vi "__Test_U8ArrayToData.vi"() -> ()   [LabVIEW 2019, in "Memory Data Access.lvlib"]
uses:
  Memory Data Access.lvlib
panel:
  out "data_Cluster":T1
  out "data_Path":path
  out "data_Str":string
  out "data_DBL":dbl
  out "data_U32":u32
  out "data_I32":i32
  out "data_Waveform":waveform(dbl)
  out "data TimeStamp":timestamp
  out "data_Bool":bool
  out "data_ArrayWav":waveform(dbl)[](array[waveform])
  out "data_ArrayDBL":dbl[](array[numeric])
  out "data_ArrayStr":string[](array[string])
  in  "Enum":T2(ring)
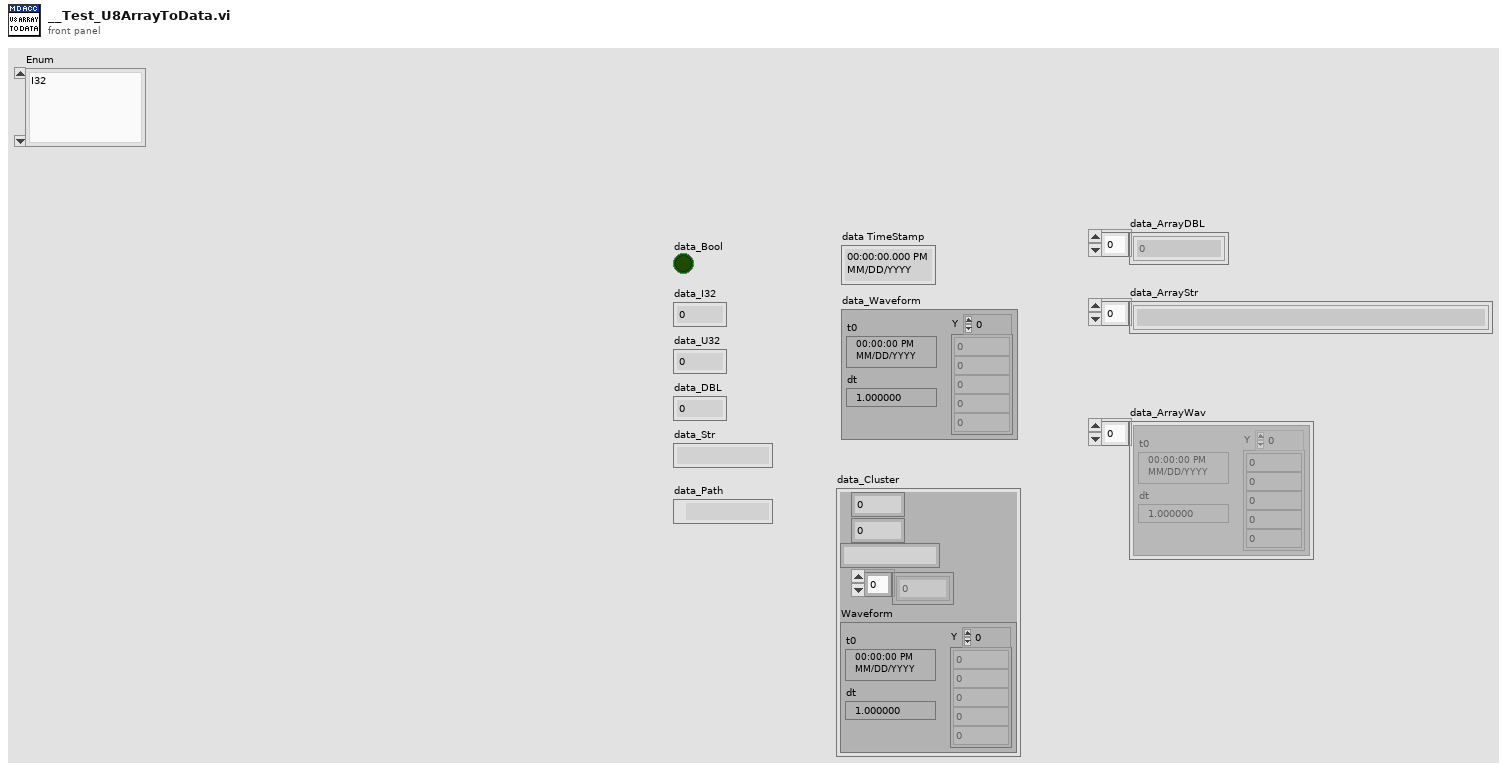
[diagram p1: front panel]
types:
  T1 = cluster{i32, dbl, string, dbl[], "Waveform":waveform(dbl)}
  T2 = enum16{"I32", "U32", "DBL", "String", "Cluster", "Array_Str", "Array_DBL", "Array_Waveform", "Bool", "TimeStamp", "Waveform", "Path"}
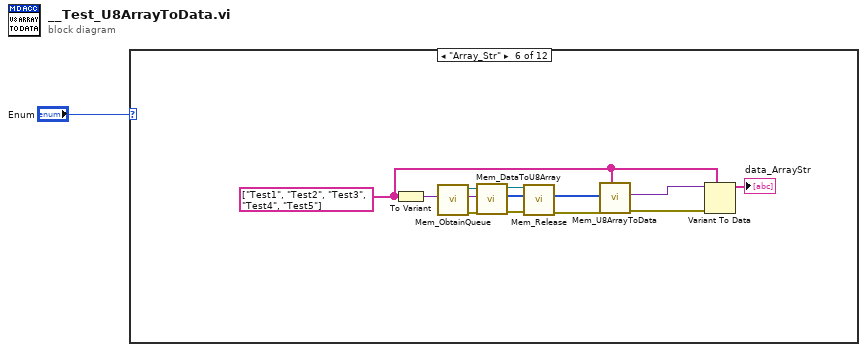
[diagram p0: block diagram]
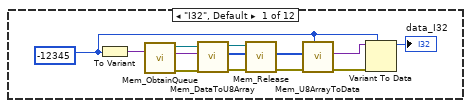
[diagram p2: hidden frame]
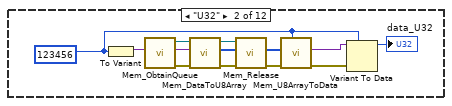
[diagram p3: hidden frame]
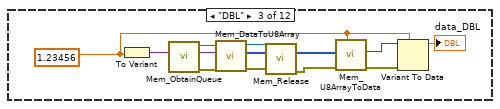
[diagram p4: hidden frame]
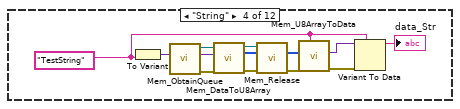
[diagram p5: hidden frame]
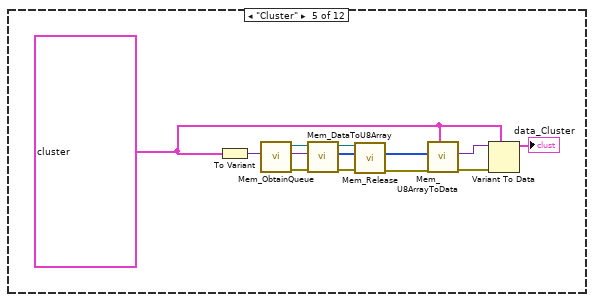
[diagram p6: hidden frame]
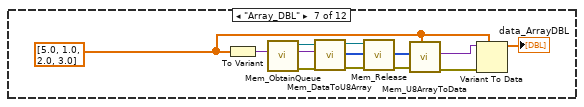
[diagram p7: hidden frame]
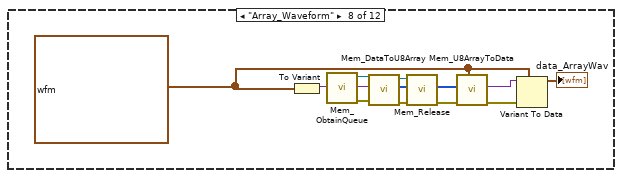
[diagram p8: hidden frame]
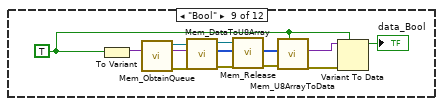
[diagram p9: hidden frame]
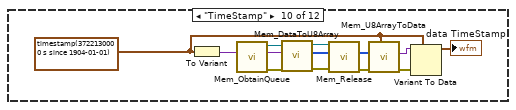
[diagram p10: hidden frame]
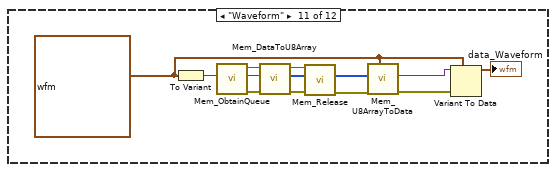
[diagram p11: hidden frame]
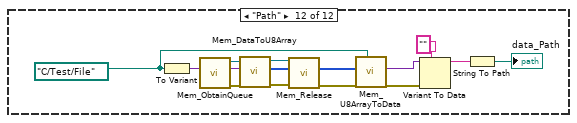
[diagram p12: hidden frame]
diagram:
  n1 = case shown="\"Array_Str\"" "Enum" {
    frame "I32", Default {
      w8 = -12345
      n2 = To Variant(anything=w8) -> (Variant=w12:variant)
      n3 = call "Mem_ObtainQueue.vi"() -> ("error out"=w6:errorcluster, "queue out"=w3:refnum<queue>)  [unwired: 10 in]
      n4 = call "Mem_DataToU8Array.vi"("error in (no error)"=w6, "Payload"=w12, "AddrQueueIn"=w3) -> ("error out"=w5:errorcluster, "ByteArray"=w11:u8[], "AddrQueueOut"=w4:refnum<queue>)  [unwired: 5 in, 1 out]
      n5 = call "Mem_Release.vi"("error in (no error)"=w5, "AddrQueueIn"=w4) -> ("error out"=w2:errorcluster)  [unwired: 9 in]
      n6 = call "Mem_U8ArrayToData.vi"("Type"=w8, "error in (no error)"=w2, "ByteArray"=w11) -> ("error out"=w10:errorcluster, "data"=w9:variant)  [unwired: 5 in, 2 out]
      n7 = Variant To Data(error in=w10, type=w8, Variant=w9) -> (data=→"data_I32":i32)  [unwired: 1 out]
    }
    frame "U32" {
      w19 = u32 123456
      n8 = To Variant(anything=w19) -> (Variant=w23:variant)
      n9 = call "Mem_ObtainQueue.vi"() -> ("error out"=w17:errorcluster, "queue out"=w16:refnum<queue>)  [unwired: 10 in]
      n10 = call "Mem_DataToU8Array.vi"("error in (no error)"=w17, "Payload"=w23, "AddrQueueIn"=w16) -> ("error out"=w15:errorcluster, "ByteArray"=w22:u8[], "AddrQueueOut"=w14:refnum<queue>)  [unwired: 5 in, 1 out]
      n11 = call "Mem_Release.vi"("error in (no error)"=w15, "AddrQueueIn"=w14) -> ("error out"=w13:errorcluster)  [unwired: 9 in]
      n12 = call "Mem_U8ArrayToData.vi"("Type"=w19, "error in (no error)"=w13, "ByteArray"=w22) -> ("error out"=w20:errorcluster, "data"=w21:variant)  [unwired: 5 in, 2 out]
      n13 = Variant To Data(error in=w20, type=w19, Variant=w21) -> (data=→"data_U32":u32)  [unwired: 1 out]
    }
    frame "DBL" {
      w30 = 1.23456
      n14 = To Variant(anything=w30) -> (Variant=w34:variant)
      n15 = call "Mem_ObtainQueue.vi"() -> ("error out"=w28:errorcluster, "queue out"=w27:refnum<queue>)  [unwired: 10 in]
      n16 = call "Mem_DataToU8Array.vi"("error in (no error)"=w28, "Payload"=w34, "AddrQueueIn"=w27) -> ("error out"=w26:errorcluster, "ByteArray"=w33:u8[], "AddrQueueOut"=w25:refnum<queue>)  [unwired: 5 in, 1 out]
      n17 = call "Mem_Release.vi"("error in (no error)"=w26, "AddrQueueIn"=w25) -> ("error out"=w24:errorcluster)  [unwired: 9 in]
      n18 = call "Mem_U8ArrayToData.vi"("Type"=w30, "error in (no error)"=w24, "ByteArray"=w33) -> ("error out"=w32:errorcluster, "data"=w31:variant)  [unwired: 5 in, 2 out]
      n19 = Variant To Data(error in=w32, type=w30, Variant=w31) -> (data=→"data_DBL":dbl)  [unwired: 1 out]
    }
    frame "String" {
      w41 = "TestString"
      n20 = To Variant(anything=w41) -> (Variant=w45:variant)
      n21 = call "Mem_ObtainQueue.vi"() -> ("error out"=w39:errorcluster, "queue out"=w38:refnum<queue>)  [unwired: 10 in]
      n22 = call "Mem_DataToU8Array.vi"("error in (no error)"=w39, "Payload"=w45, "AddrQueueIn"=w38) -> ("error out"=w37:errorcluster, "ByteArray"=w44:u8[], "AddrQueueOut"=w36:refnum<queue>)  [unwired: 5 in, 1 out]
      n23 = call "Mem_Release.vi"("error in (no error)"=w37, "AddrQueueIn"=w36) -> ("error out"=w35:errorcluster)  [unwired: 9 in]
      n24 = call "Mem_U8ArrayToData.vi"("Type"=w41, "error in (no error)"=w35, "ByteArray"=w44) -> ("error out"=w43:errorcluster, "data"=w42:variant)  [unwired: 5 in, 2 out]
      n25 = Variant To Data(error in=w43, type=w41, Variant=w42) -> (data=→"data_Str":string)  [unwired: 1 out]
    }
    frame "Cluster" {
      w52 = T1 {1245, 1.2345, "TestString", [0.0, 1.0, 2.0, 3.0], "Waveform"={"t0"=timestamp(3722126400 s since 1904-01-01), "dt"=1.0, "Y"=[1.0, 2.0, 3.0, 4.0]}}
      n26 = To Variant(anything=w52) -> (Variant=w56:variant)
      n27 = call "Mem_ObtainQueue.vi"() -> ("error out"=w50:errorcluster, "queue out"=w49:refnum<queue>)  [unwired: 10 in]
      n28 = call "Mem_DataToU8Array.vi"("error in (no error)"=w50, "Payload"=w56, "AddrQueueIn"=w49) -> ("error out"=w47:errorcluster, "ByteArray"=w55:u8[], "AddrQueueOut"=w48:refnum<queue>)  [unwired: 5 in, 1 out]
      n29 = call "Mem_Release.vi"("error in (no error)"=w47, "AddrQueueIn"=w48) -> ("error out"=w46:errorcluster)  [unwired: 9 in]
      n30 = call "Mem_U8ArrayToData.vi"("Type"=w52, "error in (no error)"=w46, "ByteArray"=w55) -> ("error out"=w53:errorcluster, "data"=w54:variant)  [unwired: 5 in, 2 out]
      n31 = Variant To Data(error in=w53, type=w52, Variant=w54) -> (data=→"data_Cluster":T1)  [unwired: 1 out]
    }
    frame "Array_Str" {
      w64 = string[] ["Test1", "Test2", "Test3", "Test4", "Test5"]
      n32 = To Variant(anything=w64) -> (Variant=w67:variant)
      n33 = call "Mem_ObtainQueue.vi"() -> ("error out"=w61:errorcluster, "queue out"=w60:refnum<queue>)  [unwired: 10 in]
      n34 = call "Mem_DataToU8Array.vi"("error in (no error)"=w61, "Payload"=w67, "AddrQueueIn"=w60) -> ("error out"=w59:errorcluster, "ByteArray"=w66:u8[], "AddrQueueOut"=w57:refnum<queue>)  [unwired: 5 in, 1 out]
      n35 = call "Mem_Release.vi"("error in (no error)"=w59, "AddrQueueIn"=w57) -> ("error out"=w58:errorcluster)  [unwired: 9 in]
      n36 = call "Mem_U8ArrayToData.vi"("Type"=w64, "error in (no error)"=w58, "ByteArray"=w66) -> ("error out"=w62:errorcluster, "data"=w65:variant)  [unwired: 5 in, 2 out]
      n37 = Variant To Data(error in=w62, type=w64, Variant=w65) -> (data=→"data_ArrayStr":string[])  [unwired: 1 out]
    }
    frame "Array_DBL" {
      w74 = dbl[] [5.0, 1.0, 2.0, 3.0]
      n38 = To Variant(anything=w74) -> (Variant=w78:variant)
      n39 = call "Mem_ObtainQueue.vi"() -> ("error out"=w72:errorcluster, "queue out"=w70:refnum<queue>)  [unwired: 10 in]
      n40 = call "Mem_DataToU8Array.vi"("error in (no error)"=w72, "Payload"=w78, "AddrQueueIn"=w70) -> ("error out"=w71:errorcluster, "ByteArray"=w77:u8[], "AddrQueueOut"=w69:refnum<queue>)  [unwired: 5 in, 1 out]
      n41 = call "Mem_Release.vi"("error in (no error)"=w71, "AddrQueueIn"=w69) -> ("error out"=w68:errorcluster)  [unwired: 9 in]
      n42 = call "Mem_U8ArrayToData.vi"("Type"=w74, "error in (no error)"=w68, "ByteArray"=w77) -> ("error out"=w75:errorcluster, "data"=w76:variant)  [unwired: 5 in, 2 out]
      n43 = Variant To Data(error in=w75, type=w74, Variant=w76) -> (data=→"data_ArrayDBL":dbl[])  [unwired: 1 out]
    }
    frame "Array_Waveform" {
      w85 = waveform(dbl)[] [{"t0"=timestamp(3705278400 s since 1904-01-01), "dt"=1.0, "Y"=[1.0, 2.0, 3.0]}, {"t0"=timestamp(3705278400 s since 1904-01-01), "dt"=1.0, "Y"=[4.0, 5.0, 6.0]}]
      n44 = To Variant(anything=w85) -> (Variant=w89:variant)
      n45 = call "Mem_ObtainQueue.vi"() -> ("error out"=w83:errorcluster, "queue out"=w81:refnum<queue>)  [unwired: 10 in]
      n46 = call "Mem_DataToU8Array.vi"("error in (no error)"=w83, "Payload"=w89, "AddrQueueIn"=w81) -> ("error out"=w82:errorcluster, "ByteArray"=w88:u8[], "AddrQueueOut"=w80:refnum<queue>)  [unwired: 5 in, 1 out]
      n47 = call "Mem_Release.vi"("error in (no error)"=w82, "AddrQueueIn"=w80) -> ("error out"=w79:errorcluster)  [unwired: 9 in]
      n48 = call "Mem_U8ArrayToData.vi"("Type"=w85, "error in (no error)"=w79, "ByteArray"=w88) -> ("error out"=w87:errorcluster, "data"=w86:variant)  [unwired: 5 in, 2 out]
      n49 = Variant To Data(error in=w87, type=w85, Variant=w86) -> (data=→"data_ArrayWav":waveform(dbl)[])  [unwired: 1 out]
    }
    frame "Bool" {
      w96 = TRUE
      n50 = To Variant(anything=w96) -> (Variant=w100:variant)
      n51 = call "Mem_ObtainQueue.vi"() -> ("error out"=w94:errorcluster, "queue out"=w93:refnum<queue>)  [unwired: 10 in]
      n52 = call "Mem_DataToU8Array.vi"("error in (no error)"=w94, "Payload"=w100, "AddrQueueIn"=w93) -> ("error out"=w92:errorcluster, "ByteArray"=w99:u8[], "AddrQueueOut"=w91:refnum<queue>)  [unwired: 5 in, 1 out]
      n53 = call "Mem_Release.vi"("error in (no error)"=w92, "AddrQueueIn"=w91) -> ("error out"=w90:errorcluster)  [unwired: 9 in]
      n54 = call "Mem_U8ArrayToData.vi"("Type"=w96, "error in (no error)"=w90, "ByteArray"=w99) -> ("error out"=w97:errorcluster, "data"=w98:variant)  [unwired: 5 in, 2 out]
      n55 = Variant To Data(error in=w97, type=w96, Variant=w98) -> (data=→"data_Bool":bool)  [unwired: 1 out]
    }
    frame "TimeStamp" {
      w107 = timestamp(3722130000 s since 1904-01-01)
      n56 = To Variant(anything=w107) -> (Variant=w111:variant)
      n57 = call "Mem_ObtainQueue.vi"() -> ("error out"=w105:errorcluster, "queue out"=w104:refnum<queue>)  [unwired: 10 in]
      n58 = call "Mem_DataToU8Array.vi"("error in (no error)"=w105, "Payload"=w111, "AddrQueueIn"=w104) -> ("error out"=w102:errorcluster, "ByteArray"=w110:u8[], "AddrQueueOut"=w103:refnum<queue>)  [unwired: 5 in, 1 out]
      n59 = call "Mem_Release.vi"("error in (no error)"=w102, "AddrQueueIn"=w103) -> ("error out"=w101:errorcluster)  [unwired: 9 in]
      n60 = call "Mem_U8ArrayToData.vi"("Type"=w107, "error in (no error)"=w101, "ByteArray"=w110) -> ("error out"=w109:errorcluster, "data"=w108:variant)  [unwired: 5 in, 2 out]
      n61 = Variant To Data(error in=w109, type=w107, Variant=w108) -> (data=→"data TimeStamp":timestamp)  [unwired: 1 out]
    }
    frame "Waveform" {
      w118 = waveform(dbl) {"t0"=timestamp(3722126400 s since 1904-01-01), "dt"=1.0, "Y"=[1.0, 2.0, 3.0, 4.0]} ("Waveform")
      n62 = To Variant(anything=w118) -> (Variant=w122:variant)
      n63 = call "Mem_ObtainQueue.vi"() -> ("error out"=w116:errorcluster, "queue out"=w115:refnum<queue>)  [unwired: 10 in]
      n64 = call "Mem_DataToU8Array.vi"("error in (no error)"=w116, "Payload"=w122, "AddrQueueIn"=w115) -> ("error out"=w114:errorcluster, "ByteArray"=w121:u8[], "AddrQueueOut"=w113:refnum<queue>)  [unwired: 5 in, 1 out]
      n65 = call "Mem_Release.vi"("error in (no error)"=w114, "AddrQueueIn"=w113) -> ("error out"=w112:errorcluster)  [unwired: 9 in]
      n66 = call "Mem_U8ArrayToData.vi"("Type"=w118, "error in (no error)"=w112, "ByteArray"=w121) -> ("error out"=w119:errorcluster, "data"=w120:variant)  [unwired: 5 in, 2 out]
      n67 = Variant To Data(error in=w119, type=w118, Variant=w120) -> (data=→"data_Waveform":waveform(dbl))  [unwired: 1 out]
    }
    frame "Path" {
      w131 = path "C:/Test/File"
      n68 = To Variant(anything=w131) -> (Variant=w135:variant)
      n69 = call "Mem_ObtainQueue.vi"() -> ("error out"=w127:errorcluster, "queue out"=w126:refnum<queue>)  [unwired: 10 in]
      n70 = call "Mem_DataToU8Array.vi"("error in (no error)"=w127, "Payload"=w135, "AddrQueueIn"=w126) -> ("error out"=w125:errorcluster, "ByteArray"=w134:u8[], "AddrQueueOut"=w124:refnum<queue>)  [unwired: 5 in, 1 out]
      n71 = call "Mem_Release.vi"("error in (no error)"=w125, "AddrQueueIn"=w124) -> ("error out"=w123:errorcluster)  [unwired: 9 in]
      n72 = call "Mem_U8ArrayToData.vi"("Type"=w131, "error in (no error)"=w123, "ByteArray"=w134) -> ("error out"=w133:errorcluster, "data"=w132:variant)  [unwired: 5 in, 2 out]
      n73 = Variant To Data(error in=w133, type="", Variant=w132) -> (data=w129:string)  [unwired: 1 out]
      n74 = String To Path(string=w129) -> (path=→"data_Path":path)
    }
  }
